vi "skil2.vi"() -> ()   [LabVIEW 2010]
uses:
  lib/Global 2.vi
panel:
  out "GPS:Status":i32(ring) items=["Uninitialized", "Antenna Error", "No Useable Satellites", "One Useable Satellite", "Two Useable Satellites", "Three Useable Satellites", "No GPS Time", "PDOP Too High", "Unuseable Satellite", "Fix Rejected", "Self Survey Complete", "Self Survey Not Complete"]
  out "files":i32 caption="осталось"
  in  "check":bool
  in  "do":bool
  out "Table":string[][](table)
  in  "stop":bool
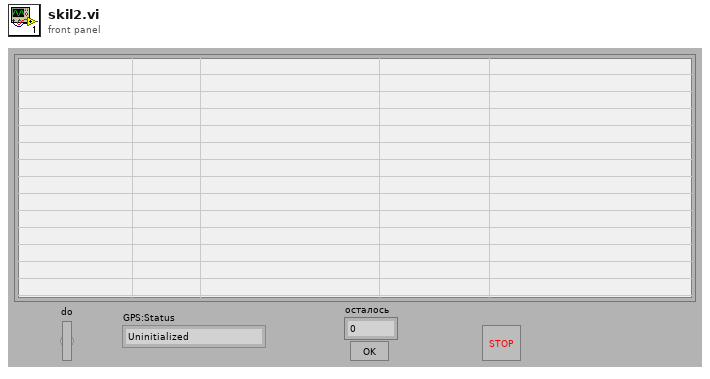
[diagram p1: front panel]
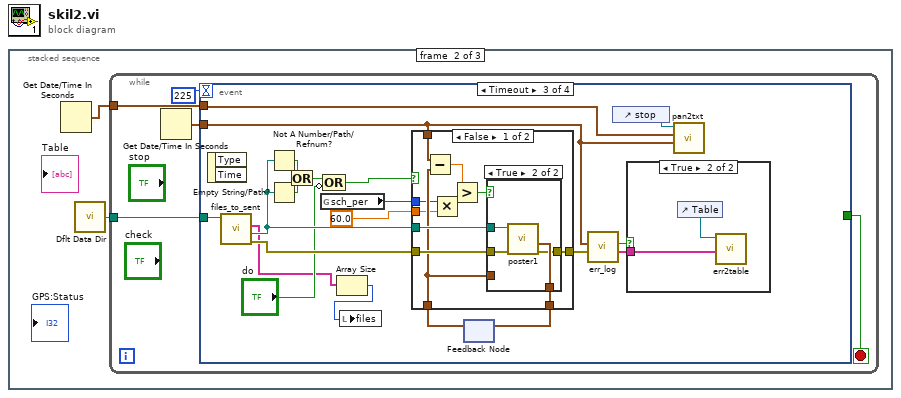
[diagram p0: block diagram]
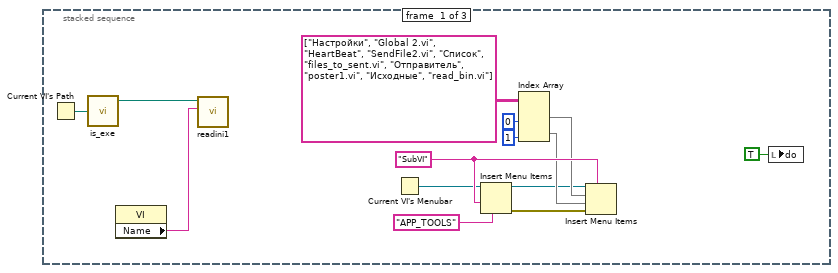
[diagram p2: hidden frame]
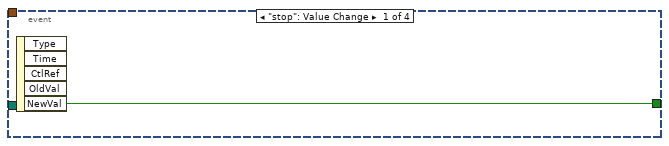
[diagram p3: hidden frame]
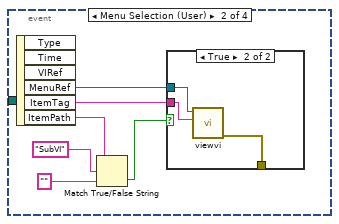
[diagram p4: hidden frame]
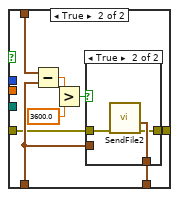
[diagram p8: hidden frame]
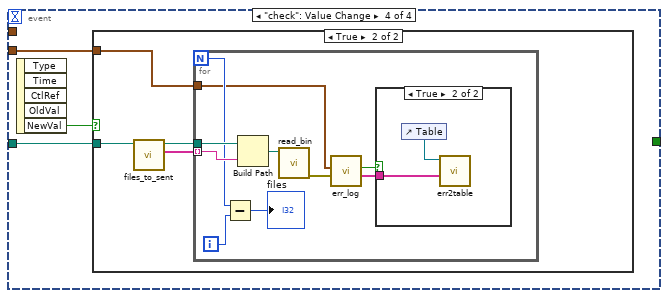
[diagram p10: hidden frame]
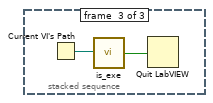
[diagram p13: hidden frame]
diagram:
  n1 = stacked-sequence {
    frame #0 {
      w11 = "SubVI"
      n2 = Current VI's Path() -> (path=w12:path)
      n3 = call "is_exe.vi"("path"=w12) -> ("ini path"=w13:path)  [unwired: 2 in, 2 out]
      n4 = property class="VI"() -> ("Name"=w14:string)  [unwired: 2 in, 2 out]
      n5 = call "readini1.vi"("section"=w14, "configuration file path"=w13) -> ()  [unwired: 3 in, 3 out]
      n6 = Current VI's Menubar() -> (w2:refnum<k9>)
      n7 = Insert Menu Items(4:"APP_TOOLS" ("after item"), 7:w11, 9:w2) -> (0:w4:errorcluster, 3:w3:refnum<k9>)  [unwired: 3 in, 1 out]
      n8 = Index Array(array=string[][] [["Настройки", "Global 2.vi"], ["HeartBeat", "SendFile2.vi"], ["Список", "files_to_sent.vi"], ["Отправитель", "poster1.vi"], ["Исходные", "read_bin.vi"]], index (col) #1=0 ("disabled index (col)"), index (col) #2=1 ("index (col)")) -> (element #1=w7:string[], element #2=w8:string[])  [unwired: 2 in]
      n9 = Insert Menu Items(5:w11, 6:w4, 7:w8, 8:w7, 9:w3) -> ()  [unwired: 1 in, 3 out]
      n10 = local write "do"(TRUE ("do")) -> ()
    }
    frame #1 {
      n11 = Get Date/Time In Seconds() -> (seconds since 1Jan1904=w15:timestamp)
      n12 = call <vilib>:"Dflt Data Dir.vi"() -> ("App:Default Data Directory"=w16:path)
      n13 = while {
        tunnel: w16 -> [w19]
        tunnel: w15 -> [w17]
        stop <- w21 stop-if-true
        n14 = Get Date/Time In Seconds() -> (seconds since 1Jan1904=w18:timestamp)
        n15 = event shown="[2] Timeout" {
          selector: _ -> [_ _ _ _]
          dyn-events: _ -> [_ _ _ _]
          timeout: 225 -> [_ _ _ _]
          tunnel: [w22 _ _ _] -> w21
          tunnel: w19 -> [_ _ w45 w85]
          tunnel: w18 -> [_ _ w38 w84]
          tunnel: w17 -> [_ _ w32 _]
          event "stop": Value Change {
            n16 = event-data() -> ("NewVal"=w22:bool)  [unwired: 1 in, 4 out]
          }
          event Menu Selection (User) {
            n17 = event-data() -> ("MenuRef"=w28:refnum<k9>, "ItemTag"=w23:string, "ItemPath"=w25:string)  [unwired: 1 in, 3 out]
            n18 = Match True/False String(2:"" ("false string"), 3:"SubVI" ("true string"), 4:w25) -> (0:w24:bool)  [unwired: 1 out]
            n19 = case shown="True" w24 {
              tunnel: w28 -> [_ w31]
              tunnel: [_ w30] -> _
              tunnel: w23 -> [_ w29]
              frame False {
              }
              frame True {
                n20 = call "viewvi.vi"("item tag"=w29, "menu reference"=w31) -> ("error out"=w30:errorcluster)  [unwired: 5 in]
              }
            }
          }
          event Timeout {
            n21 = event-data() -> ()  [unwired: 1 in, 2 out]
            n22 = call "files_to_sent.vi"("Directory"=w45) -> ("error IO"=w47:errorcluster, "file_1 path"=w46:path, "names"=w36:string[])  [unwired: 3 in, 1 out]
            n23 = Not A Number/Path/Refnum?(number/path/refnum=w46) -> (NaN/Path/Refnum?=w50:bool)
            n24 = Empty String/Path?(string/path=w46) -> (empty?=w51:bool)
            n25 = Or(x=w50, y=w51) -> (x .or. y?=w41:bool)
            n26 = global read "Global 2.vi" "sch_per"() -> (w37:i32)
            n27 = Compound Arithmetic op=OR(w41, invert "do") -> (w40:bool)
            n28 = Array Size(array=w36) -> (size(s)=w35:i32)
            n29 = local write "files"(w35) -> ()
            n30 = feedback #1() -> (w49:timestamp)  [unwired: 1 in]
            n31 = case shown="False" w40 {
              tunnel: w46 -> [w64 _]
              tunnel: w47 -> [w62 w72]
              tunnel: [w63 w75] -> w48
              tunnel: w49 -> [w57 w74]
              tunnel: [w61 w73] -> w44
              tunnel: w38 -> [w60 w71]
              tunnel: w37 -> [w56 _]
              tunnel: 60.0 -> [w54 _]
              frame False {
                n32 = Subtract(x=w60, y=w57) -> (x-y=w59:dbl)
                n33 = Multiply(x=w56, y=w54) -> (x*y=w55:dbl)
                n34 = Greater?(x=w59, y=w55) -> (0:w58:bool)
                n35 = case shown="True" w58 {
                  tunnel: w64 -> [_ w70]
                  tunnel: [w65 w69] -> w63
                  tunnel: w62 -> [w66 w68]
                  tunnel: [w66 w67] -> w61
                  tunnel: w57 -> [w65 _]
                  frame False {
                  }
                  frame True {
                    n36 = call "poster1.vi"("error in"=w68, "file path"=w70) -> ("error out"=w67:errorcluster, "last ses time"=w69:timestamp)  [unwired: 2 in, 2 out]
                  }
                }
              }
              frame True {
                n37 = Subtract(x=w71, y=w74) -> (x-y=w78:dbl)
                n38 = Greater?(x=w78, y=3600.0) -> (0:w76:bool)
                n39 = case shown="True" w76 {
                  tunnel: [w80 w83] -> w75
                  tunnel: w74 -> [w80 _]
                  tunnel: [w79 w82] -> w73
                  tunnel: w72 -> [w79 w81]
                  frame False {
                  }
                  frame True {
                    n40 = call "SendFile2.vi"("error in"=w81) -> ("error out"=w82:errorcluster, "last ses time"=w83:timestamp)  [unwired: 5 in]
                  }
                }
              }
            }
            n41 = feedback-in #1(w48) -> ()
            n42 = call "err_log.vi"("error In"=w44, "time stamp"=w38) -> ("err_table"=w43:string[], "do?"=w39:bool)  [unwired: 4 in]
            n43 = control-ref of="stop"() -> (w33:refnum<vi>)
            n44 = case shown="True" w39 {
              tunnel: w43 -> [_ w53]
              frame False {
              }
              frame True {
                n45 = control-ref of="Table"() -> (w52:refnum<vi>)
                n46 = call "err2table.vi"("err_table"=w53, "Tbl Refnum"=w52) -> ()  [unwired: 6 in]
              }
            }
            n47 = call "pan2txt.vi"("seconds since 1Jan1904"=w38, "started"=w32, "stop button"=w33) -> ()  [unwired: 5 in]
          }
          event "check": Value Change {
            n48 = event-data() -> ("NewVal"=w86:bool)  [unwired: 1 in, 4 out]
            n49 = case shown="True" w86 {
              tunnel: w85 -> [_ w90]
              tunnel: w84 -> [_ w87]
              frame False {
              }
              frame True {
                n50 = call "files_to_sent.vi"("Directory"=w90) -> ("names"=w89:string[], "directory dup"=w88:path)  [unwired: 3 in, 2 out]
                n51 = for {
                  N -> [w96]
                  tunnel: w89 -> [w99] mode=indexing
                  tunnel: w88 -> [w100]
                  tunnel: w87 -> [w94]
                  i -> [w97]
                  n52 = Subtract(x=w96, y=w97) -> (x-y=→"files":i32)
                  n53 = Build Path(base path=w100, name or relative path=w99) -> (appended path=w98:path)
                  n54 = call "read_bin.vi"("datalog path"=w98) -> ("error out"=w92:errorcluster)  [unwired: 3 in, 3 out]
                  n55 = call "err_log.vi"("error In"=w92, "time stamp"=w94) -> ("err_table"=w93:string[], "do?"=w91:bool)  [unwired: 4 in]
                  n56 = case shown="True" w91 {
                    tunnel: w93 -> [_ w102]
                    frame False {
                    }
                    frame True {
                      n57 = control-ref of="Table"() -> (w101:refnum<vi>)
                      n58 = call "err2table.vi"("err_table"=w102, "Tbl Refnum"=w101) -> ()  [unwired: 6 in]
                    }
                  }
                }
              }
            }
          }
        }
      }
    }
    frame #2 {
      n59 = Current VI's Path() -> (path=w103:path)
      n60 = call "is_exe.vi"("path"=w103) -> ("exe?"=w104:bool)  [unwired: 2 in, 2 out]
      n61 = Quit LabVIEW(quit? (T)=w104) -> ()
    }
  }
